vi "SetTemp.vi"(7 "pause?":bool=TRUE, 8 "error in":errorcluster, 10 "temp":i32=20 caption="Temperature", 11 "camera.nit in":refnum<class "camera.lvclass">) -> (0 "error out":errorcluster)   [LabVIEW 2020, in "camera.lvclass"]
uses:
  camera.lvclass
  7982a402-e577-4aaa-ab54-7a3c9b5797b6.vi
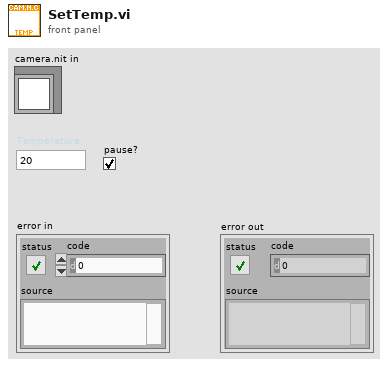
[diagram p1: front panel]
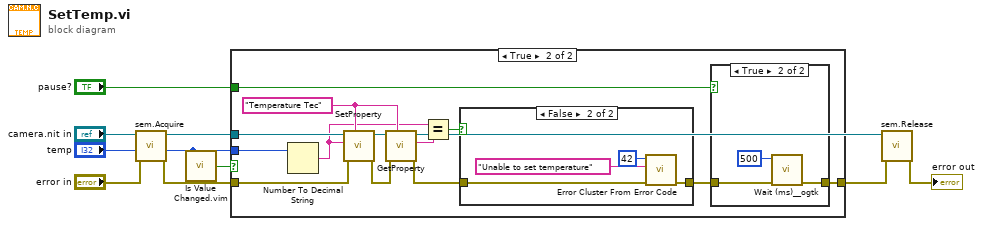
[diagram p0: block diagram]
diagram:
  n1 = call "sem.Acquire.vi"("error in"="error in", "camera.nit in"="camera.nit in") -> ("error out"=w7:errorcluster)  [unwired: 9 in]
  n2 = call "Is Value Changed.vim"("value"="temp") -> ("changed or first call?"=w1:bool)
  n3 = case shown="True" w1 {
    tunnel: "temp" -> [_ w17]
    tunnel: w7 -> [w9 w14]
    tunnel: "camera.nit in" -> [_ w13]
    tunnel: "pause?" -> [_ w12]
    tunnel: [w9 w10] -> w3
    frame False {
    }
    frame True {
      w19 = "Temperature Tec" ("pPrp")
      n4 = Number To Decimal String(number=w17) -> (decimal integer string=w16:string)  [unwired: 1 in]
      n5 = call-dynamic "SetProperty.vi"("Property"=w19, "error in"=w14, "Value"=w16, "camera.nit in"=w13) -> ("error out"=w18:errorcluster)  [unwired: 7 in]
      n6 = call-dynamic "GetProperty.vi"("Property"=w19, "error in"=w18, "camera.nit in"=w13) -> ("error out"=w15:errorcluster, "value"=w20:string)  [unwired: 7 in]
      n7 = Equal?(x=w16, y=w20) -> (x = y?=w21:bool)
      n8 = case shown="False" w21 {
        tunnel: w15 -> [w26 w30]
        tunnel: [w26 w28] -> w11
        frame True {
        }
        frame False {
          n9 = call <vilib>:"Error Cluster From Error Code.vi"("error in (no error)"=w30, "error message (\"\")"="Unable to set temperature" ("error message (\"\")"), "error code (0)"=42) -> ("error out"=w28:errorcluster)  [unwired: 6 in]
        }
      }
      n10 = case shown="True" w12 {
        tunnel: w11 -> [w22 w25]
        tunnel: [w22 w24] -> w10
        frame False {
        }
        frame True {
          n11 = call <userlib>:"Wait (ms)__ogtk.vi"("error in (no error)"=w25, "milliseconds to wait"=u32 500) -> ("error out"=w24:errorcluster)  [unwired: 8 in, 1 out]
        }
      }
    }
  }
  n12 = call "sem.Release.vi"("error in"=w3, "camera.nit in"="camera.nit in") -> ("error out"=→"error out":errorcluster)  [unwired: 9 in]
